vi "Set PSU Inhibit.vi"(4 "error in":errorcluster, 6 "On/Off":bool) -> (0 "error out":errorcluster)   [LabVIEW 2015]
uses:
  <vilib>/DAQmx/write.llb/DAQmx Write (Digital Bool 1Line 1Point).vi
  <vilib>/DAQmx/miscellaneous.llb/DAQmx Fill In Error Info.vi
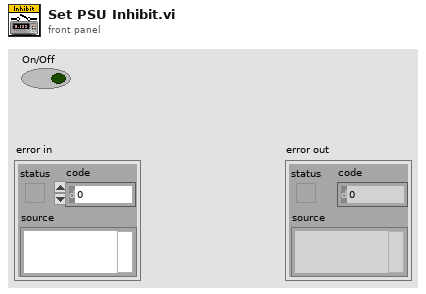
[diagram p1: front panel]
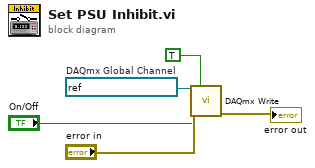
[diagram p0: block diagram]
diagram:
  w5 = refnum<k21> "DO3 PSU Inhibit"  # DAQmx Global Channel
  n1 = call-poly <vilib>:"DAQmx Write.vi"("task/channels in"=w5, "auto start"=TRUE, "data"="On/Off", "error in"="error in") -> ("error out"=→"error out":errorcluster)  [unwired: 9 in, 2 out]
